vi "cameraCalibration.vi"() -> ()   [LabVIEW 2020]
panel:
  out "output 2":dbl
  out "output 1":dbl
  in  "calibration file":path
  in  "Recalibrate":bool
  out "F_y":dbl
  out "F_x":dbl
  in  "Image x coordinate (px)":dbl=1179.0
  in  "Image y coordinate (px)":dbl=800.0
  in  "Image height (px)":dbl=1080.0
  in  "Image width (px)":dbl=1920.0
  in  "Lateral y distance (m)":dbl=-1.03
  in  "Longitudinal x distance (m)":dbl=7.03
  in  "Camera height (m)":dbl=1.36
  # "Fill in all values below of an aribtrary object in the image with known coordinates, run the VI and press the button below to recalibrate the main program for the current camera and its position.\n\nAs long as the aspect ratio and field of view stay the same, the program does not need to be recalibrated for different camera resolutions."
  # "Image coordinates"
  # "Real-life coordinates"
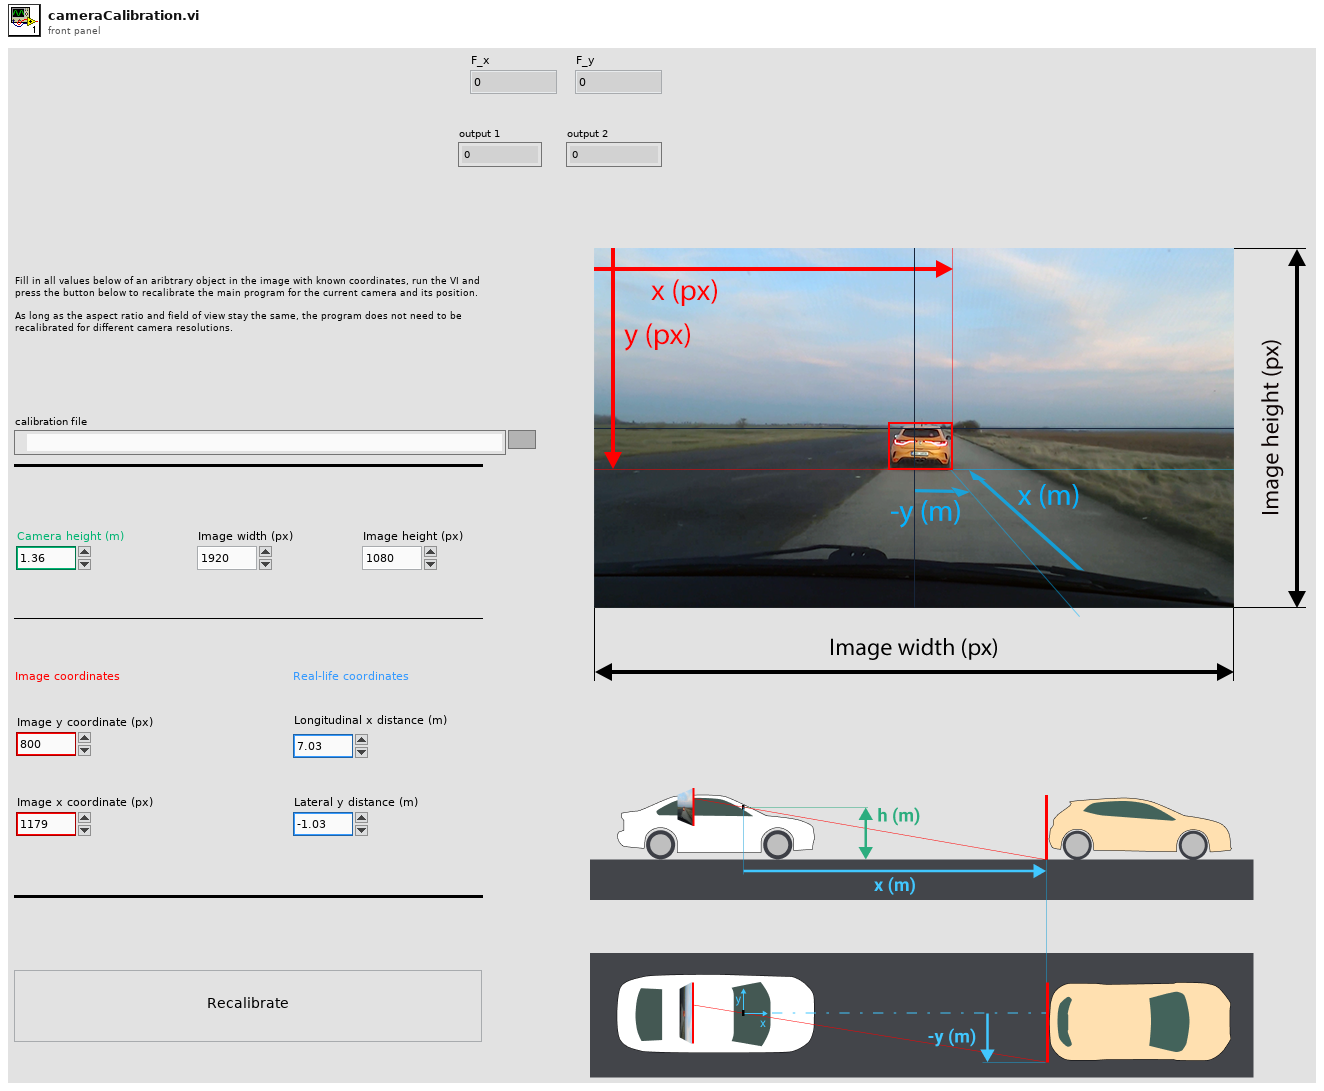
[diagram p1: front panel]
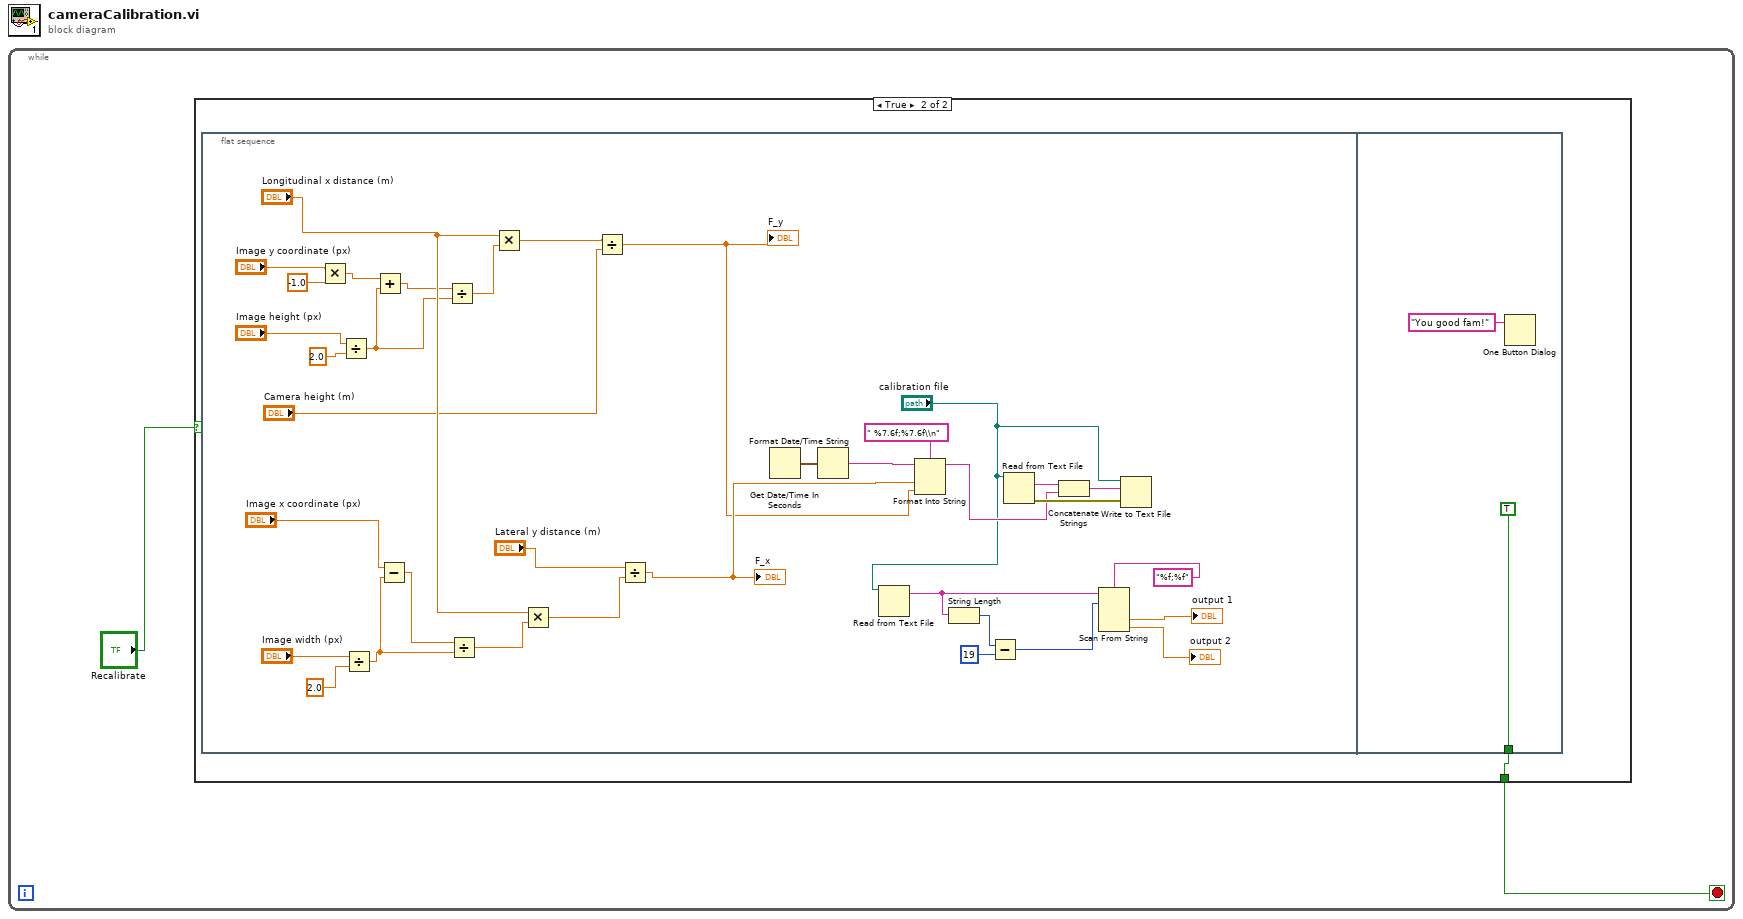
[diagram p0: block diagram]
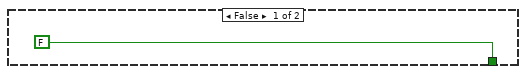
[diagram p2: hidden frame]
diagram:
  n1 = while {
    stop <- w1 stop-if-true
    n2 = case shown="True" "Recalibrate" {
      tunnel: [FALSE w4] -> w1
      frame False {
      }
      frame True {
        n3 = flat-sequence {
          tunnel: [TRUE] -> w4
          frame #0 {
            n4 = Multiply(x="Image y coordinate (px)", y=-1.0) -> (x*y=w26:dbl)
            n5 = Divide(x="Image height (px)", y=2.0) -> (x/y=w27:dbl)
            n6 = Divide(x="Image width (px)", y=2.0) -> (x/y=w22:dbl)
            n7 = Add(x=w26, y=w27) -> (x+y=w25:dbl)
            n8 = Subtract(x="Image x coordinate (px)", y=w22) -> (x-y=w24:dbl)
            n9 = Divide(x=w25, y=w27) -> (x/y=w40:dbl)
            n10 = Divide(x=w24, y=w22) -> (x/y=w39:dbl)
            n11 = Multiply(x="Longitudinal x distance (m)", y=w40) -> (x*y=w35:dbl)
            n12 = Multiply(x="Longitudinal x distance (m)", y=w39) -> (x*y=w37:dbl)
            n13 = Divide(x=w35, y="Camera height (m)") -> (x/y=w13:dbl)
            "F_y" <- w13
            n14 = Divide(x="Lateral y distance (m)", y=w37) -> (x/y=w14:dbl)
            "F_x" <- w14
            n15 = Get Date/Time In Seconds() -> (seconds since 1Jan1904=w21:timestamp)
            n16 = Format Date/Time String(seconds (now)=w21) -> (date/time string=w17:string)  [unwired: 2 in]
            n17 = Read from Text File(file (use dialog)="calibration file") -> (text=w9:string)  [unwired: 3 in, 3 out]
            n18 = Format Into String(format string=" %7.6f;%7.6f\\n", initial string=w17, w14, w13) -> (resulting string=w16:string)  [unwired: 1 in, 1 out]
            n19 = String Length(string=w9) -> (length=w8:i32)
            n20 = Subtract(x=w8, y=19) -> (x-y=w6:i32)
            n21 = Read from Text File(file (use dialog)="calibration file") -> (text=w18:string, error out=w19:errorcluster)  [unwired: 3 in, 2 out]
            n22 = Concatenate Strings(w18, w16) -> (w15:string)
            n23 = Scan From String(format string="%f;%f", input string=w9, initial scan location=w6) -> (output 1=→"output 1":dbl, output 2=→"output 2":dbl)  [unwired: 3 in, 3 out]
            n24 = Write to Text File(file (use dialog)="calibration file", text=w15, error in=w19) -> ()  [unwired: 1 in, 3 out]
          }
          frame #1 {
            n25 = One Button Dialog(message="You good fam!") -> ()  [unwired: 1 in, 1 out]
          }
        }
      }
    }
  }
